vi "INA219 Read Measurements.vi"(8 "error in (no error)":errorcluster, 9 "INA219 Config Options":T1={"I2C"={"Slave Address"=64, "Channel"=0}, "Reset bit"=0, "Bus Voltage Range"=1, "PGA/Shunt Voltage Gain"=3, "Bus Voltage ADC Settings"=8, "Shunt Voltage ADC Settings"=3, "Mode"=7, "Calibration Value"=4096, "Online"=FALSE, "Shunt Resistor"=0.1} {"Shunt Resistor" format="%#_g ohm"; "I2C"."Slave Address" format="%.0x"; "Calibration Value" format="%.0x"; "Mode" items=["Power Down", "Shunt Voltage, Triggered", "Bus Voltage, Triggered", "Shunt & Bus, Triggered", "ADC Off (Disabled)", "Shunt Voltage, Continuous", "Bus Voltage, Continuous", "Shunt & Bus Voltage, Continuous"]; "Shunt Voltage ADC Settings" items=["9-bit, 84us conversion time"=0, "10-bit, 148us conversion time"=1, "11-bit, 276us conversion time"=2, "12-bit, 532us conversion time"=3, "1x12-bit, 532us conversion time"=8, "2x12-bit averaged, 1.06ms conversion time"=9, "4x12-bit averaged, 2.13ms conversion time"=10, "8x12-bit averaged, 4.26ms conversion time"=11, "16x12-bit averaged, 8.51ms conversion time"=12, "32x12-bit averaged, 17.02ms conversion time"=13, "64x12-bit averaged, 34.05ms conversion time"=14, "128x12-bit averaged, 68.10ms conversion time"=15]; "Bus Voltage ADC Settings" items=["9-bit, 84us conversion time"=0, "10-bit, 148us conversion time"=1, "11-bit, 276us conversion time"=2, "12-bit, 532us conversion time"=3, "1x12-bit, 532us conversion time"=8, "2x12-bit averaged, 1.06ms conversion time"=9, "4x12-bit averaged, 2.13ms conversion time"=10, "8x12-bit averaged, 4.26ms conversion time"=11, "16x12-bit averaged, 8.51ms conversion time"=12, "32x12-bit averaged, 17.02ms conversion time"=13, "64x12-bit averaged, 34.05ms conversion time"=14, "128x12-bit averaged, 68.10ms conversion time"=15]; "PGA/Shunt Voltage Gain" items=["Gain 1, +/-40mV", "Gain 2, +/-80mV", "Gain 3, +/-160mV", "Gain 4, +/-320mV"]; "Bus Voltage Range" items=["0-16V Range", "0-32V Range"]; "Reset bit" items=["Do Not Reset", "Reset"]}, 11 "LINX Resource in":T3) -> (0 "error out":errorcluster, 1 "INA219 Config Options":T1={"I2C"={"Slave Address"=64, "Channel"=0}, "Reset bit"=0, "Bus Voltage Range"=1, "PGA/Shunt Voltage Gain"=3, "Bus Voltage ADC Settings"=8, "Shunt Voltage ADC Settings"=3, "Mode"=7, "Calibration Value"=4096, "Online"=FALSE, "Shunt Resistor"=0.1} {"Shunt Resistor" format="%#_g ohm"; "I2C"."Slave Address" format="%.0x"; "Calibration Value" format="%.0x"; "Mode" items=["Power Down", "Shunt Voltage, Triggered", "Bus Voltage, Triggered", "Shunt & Bus, Triggered", "ADC Off (Disabled)", "Shunt Voltage, Continuous", "Bus Voltage, Continuous", "Shunt & Bus Voltage, Continuous"]; "Shunt Voltage ADC Settings" items=["9-bit, 84us conversion time"=0, "10-bit, 148us conversion time"=1, "11-bit, 276us conversion time"=2, "12-bit, 532us conversion time"=3, "1x12-bit, 532us conversion time"=8, "2x12-bit averaged, 1.06ms conversion time"=9, "4x12-bit averaged, 2.13ms conversion time"=10, "8x12-bit averaged, 4.26ms conversion time"=11, "16x12-bit averaged, 8.51ms conversion time"=12, "32x12-bit averaged, 17.02ms conversion time"=13, "64x12-bit averaged, 34.05ms conversion time"=14, "128x12-bit averaged, 68.10ms conversion time"=15]; "Bus Voltage ADC Settings" items=["9-bit, 84us conversion time"=0, "10-bit, 148us conversion time"=1, "11-bit, 276us conversion time"=2, "12-bit, 532us conversion time"=3, "1x12-bit, 532us conversion time"=8, "2x12-bit averaged, 1.06ms conversion time"=9, "4x12-bit averaged, 2.13ms conversion time"=10, "8x12-bit averaged, 4.26ms conversion time"=11, "16x12-bit averaged, 8.51ms conversion time"=12, "32x12-bit averaged, 17.02ms conversion time"=13, "64x12-bit averaged, 34.05ms conversion time"=14, "128x12-bit averaged, 68.10ms conversion time"=15]; "PGA/Shunt Voltage Gain" items=["Gain 1, +/-40mV", "Gain 2, +/-80mV", "Gain 3, +/-160mV", "Gain 4, +/-320mV"]; "Bus Voltage Range" items=["0-16V Range", "0-32V Range"]; "Reset bit" items=["Do Not Reset", "Reset"]}, 2 "Measurements":T2 {"Current" format="%#.3g A"; "Power" format="%#.3g W"; "Shunt Voltage" format=" %#.3g V"; "Bus Voltage" format="%#.3g V"; "Voltage (Total)" format="%#.3g V"}, 3 "LINX Resource":T3)   [LabVIEW 2014]
uses:
  <vilib>/MakerHub/LINX/Private/Type Defs/LINX Ref.ctl
  <vilib>/MakerHub/LINX/Private/Type Defs/Platform.ctl
  <vilib>/MakerHub/LINX/Private/Type Defs/Interface.ctl
  <vilib>/MakerHub/LINX/Private/Device/Type Defs/LINX Device Config.ctl
  <vilib>/MakerHub/LINX/Private/Device/Type Defs/TCP Config.ctl
  <vilib>/MakerHub/LINX/Private/Device/Type Defs/Channels.ctl
  INA219 Measurements.ctl
  INA219 Config Options.ctl
  <vilib>/MakerHub/LINX/LMH-LINX.lvlib
  <vilib>/MakerHub/LINX/Private/Device/Device.lvlib
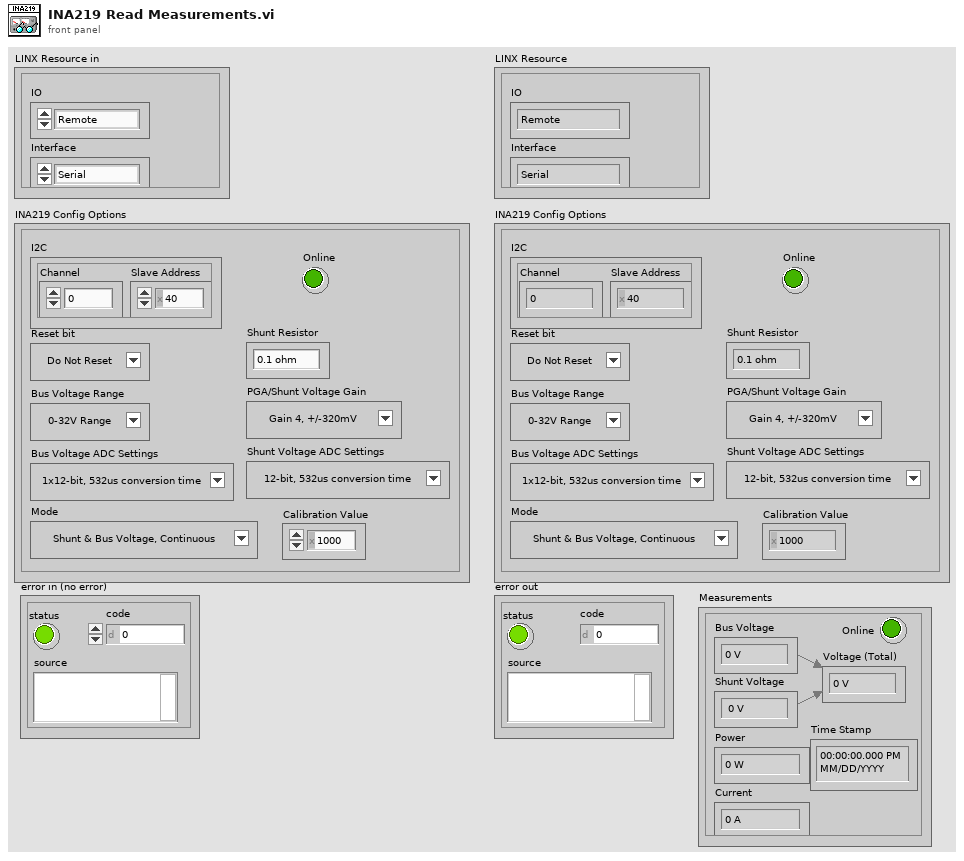
[diagram p1: front panel]
types:
  T1 = typedef "INA219 Config Options.ctl" = cluster{"I2C":cluster{"Slave Address":u8, "Channel":u8}, "Reset bit":u8, "Bus Voltage Range":u8, "PGA/Shunt Voltage Gain":u8, "Bus Voltage ADC Settings":u8, "Shunt Voltage ADC Settings":u8, "Mode":u8, "Calibration Value":u16, "Online":bool, "Shunt Resistor":dbl}
  T2 = typedef "INA219 Measurements.ctl" = cluster{"Voltage (Total)":dbl, "Bus Voltage":dbl, "Shunt Voltage":dbl, "Power":dbl, "Current":dbl, "Online":bool, "Time Stamp":timestamp}
  T3 = typedef "LMH-LINX.lvlib/LINX Ref.ctl" = cluster{"IO":T4, "Interface":T5, "LINX Device Config":T6}
  T4 = typedef "LMH-LINX.lvlib/Platform.ctl" = enum16{"Remote", "Local"}
  T5 = typedef "LMH-LINX.lvlib/Interface.ctl" = enum16{"Serial", "TCP"}
  T6 = typedef "LMH-LINX.lvlib/Device.lvlib/LINX Device Config.ctl" = cluster{"Interface":T5, "COM Port":refnum<visa-resource-name>, "TCP Configuration":T7, "Device Family":u8, "Device ID":u8, "Device Name":string, "TCP Ref":refnum<k5>, "Channels":T8}
  T7 = typedef "LMH-LINX.lvlib/Device.lvlib/TCP Config.ctl" = cluster{"IP Address":string, "Port":u16}
  T8 = typedef "LMH-LINX.lvlib/Channels.ctl" = cluster{"DI":u8[], "DO":u8[], "AI":u8[], "AO":u8[], "PWM":u8[], "QE":u8[], "UART":u8[], "I2C 2":u8[], "SPI":u8[], "CAN":u8[], "Servo":u8[], "AI Ref (V)":dbl, "AI Resolution (Bits)":u8, "AO Ref (V)":dbl, "AO Resolution (Bits)":u8}
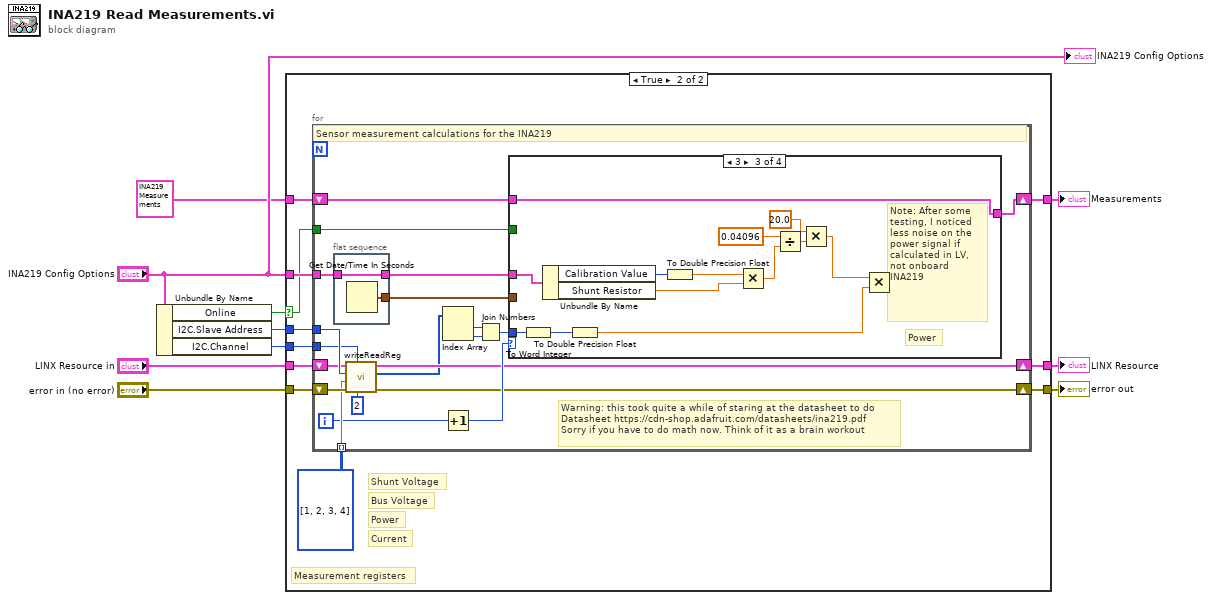
[diagram p0: block diagram]
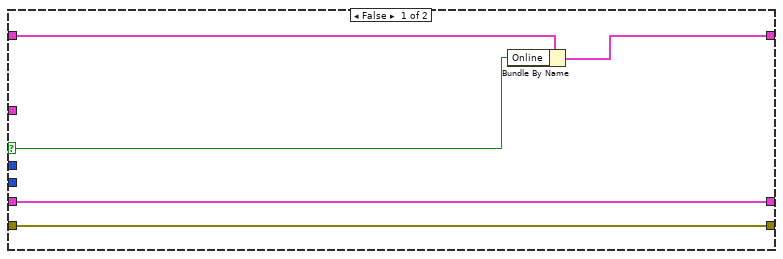
[diagram p2: hidden frame]
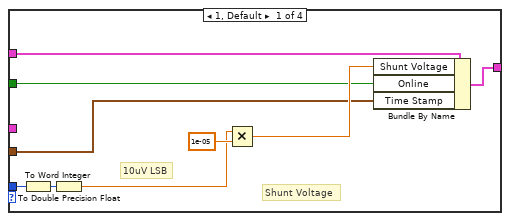
[diagram p3: hidden frame]
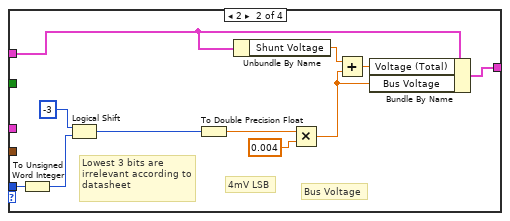
[diagram p4: hidden frame]
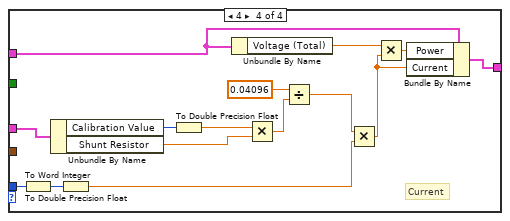
[diagram p5: hidden frame]
diagram:
  n1 = Unbundle By Name("INA219 Config Options") -> ("Online"=w1:bool, "I2C.Slave Address"=w4:u8, "I2C.Channel"=w5:u8)
  n2 = case shown="True" w1 {
    selector: w1 -> [w11 w16]
    tunnel: "error in (no error)" -> [w14 w26]
    tunnel: "LINX Resource in" -> [w15 w25]
    tunnel: [w14 w24] -> w8
    tunnel: [w15 w23] -> w7
    tunnel: [w12 w21] -> w6
    tunnel: w5 -> [_ w20]
    tunnel: w4 -> [_ w19]
    tunnel: "INA219 Config Options" -> [_ w18]
    tunnel: T2 {"Voltage (Total)"=0.0, "Bus Voltage"=0.0, "Shunt Voltage"=0.0, "Power"=0.0, "Current"=0.0, "Online"=FALSE, "Time Stamp"=timestamp(0 s since 1904-01-01)} ("Measurements") -> [w13 w17]
    frame False {
      n3 = Bundle By Name(cluster=w13, "Online"=w11) -> (w12:T2)
    }
    frame True {
      # "Measurement registers"
      # "Current"
      # "Power"
      # "Bus Voltage"
      # "Shunt Voltage"
      n4 = for {
        tunnel: w19 -> [w46]
        tunnel: w20 -> [w45]
        shift-right: [w32] -> w24
        shift-left: w26 -> [w44]
        shift-right: [w33] -> w23
        shift-left: w25 -> [w43]
        tunnel: u8[][] [[1], [2], [3], [4]] ("Data") -> [w42] mode=indexing
        tunnel: w18 -> [w29]
        shift-right: [w35] -> w21
        shift-left: w17 -> [w36]
        tunnel: w16 -> [w30]
        i -> [w39]
        # "Warning: this took quite a while of staring at the datasheet to do\nDatasheet https://cdn-shop.adafruit.com/datasheets/ina219.pdf\nSorry if you have to do math now. Think of it as a brain workout"
        # "Sensor measurement calculations for the INA219"
        n5 = flat-sequence {
          tunnel: w29 -> [w48]
          tunnel: [w48] -> w28
          tunnel: [w47] -> w27
          frame #0 {
            n6 = Get Date/Time In Seconds() -> (seconds since 1Jan1904=w47:timestamp)
          }
        }
        n7 = call "writeReadReg.vi"("Bytes To Read"=u8 2, "I2C Channel"=w45, "error in"=w44, "Data"=w42, "I2C Slave Address"=w46, "LINX Resource in"=w43) -> ("error out"=w32:errorcluster, "Bytes Read"=w31:u8[], "LINX Resource out"=w33:T3)  [unwired: 3 in]
        n8 = Index Array(array=w31) -> (element #1=w40:u8, element #2=w41:u8)  [unwired: 2 in]
        n9 = Increment(x=w39) -> (x+1=w38:i32)
        n10 = Join Numbers(hi=w40, lo=w41) -> ((hi.lo)=w37:u16)
        n11 = case shown="3" w38 {
          tunnel: w37 -> [w56 w62 w80 w95]
          tunnel: w28 -> [_ _ w81 w96]
          tunnel: w36 -> [w57 w67 w70 w86]
          tunnel: [w53 w68 w70 w93] -> w35
          tunnel: w30 -> [w50 _ _ _]
          tunnel: w27 -> [w49 _ _ _]
          frame 1, Default {
            # "10uV LSB"
            # "Shunt Voltage"
            n12 = To Word Integer(number=w56) -> (16bit integer=w54:i16)
            n13 = To Double Precision Float(number=w54) -> (double precision float=w51:dbl)
            n14 = Multiply(x=w51, y=1e-05) -> (x*y=w55:dbl)
            n15 = Bundle By Name(cluster=w57, "Shunt Voltage"=w55, "Online"=w50, "Time Stamp"=w49) -> (w53:T2)
          }
          frame 2 {
            # "Lowest 3 bits are irrelevant according to datasheet"
            # "4mV LSB"
            # "Bus Voltage"
            n16 = To Unsigned Word Integer(number=w62) -> (unsigned 16bit integer=w61:u16)
            n17 = Logical Shift(y=i16 -3, x=w61) -> (x << y=w59:u16)
            n18 = To Double Precision Float(number=w59) -> (double precision float=w63:dbl)
            n19 = Unbundle By Name(w67) -> ("Shunt Voltage"=w65:dbl)
            n20 = Multiply(x=w63, y=0.004) -> (x*y=w66:dbl)
            n21 = Add(x=w65, y=w66) -> (x+y=w58:dbl)
            n22 = Bundle By Name(cluster=w67, "Voltage (Total)"=w58, "Bus Voltage"=w66) -> (w68:T2)
          }
          frame 3 {
            # "Note: After some testing, I noticed less noise on the power signal if calculated in LV, not onboard INA219"
            # "Power"
            n23 = To Word Integer(number=w80) -> (16bit integer=w75:i16)
            n24 = Unbundle By Name(w81) -> ("Calibration Value"=w76:u16, "Shunt Resistor"=w69:dbl)
            n25 = To Double Precision Float(number=w75) -> (double precision float=w74:dbl)
            n26 = To Double Precision Float(number=w76) -> (double precision float=w77:dbl)
            n27 = Multiply(x=w77, y=w69) -> (x*y=w79:dbl)
            n28 = Divide(x=0.04096, y=w79) -> (x/y=w72:dbl)
            n29 = Multiply(x=20.0, y=w72) -> (x*y=w73:dbl)
            n30 = Multiply(x=w73, y=w74) -> ()  [unwired: 1 out]
          }
          frame 4 {
            # "Current"
            n31 = To Word Integer(number=w95) -> (16bit integer=w94:i16)
            n32 = Unbundle By Name(w96) -> ("Calibration Value"=w90:u16, "Shunt Resistor"=w82:dbl)
            n33 = To Double Precision Float(number=w94) -> (double precision float=w88:dbl)
            n34 = To Double Precision Float(number=w90) -> (double precision float=w89:dbl)
            n35 = Unbundle By Name(w86) -> ("Voltage (Total)"=w84:dbl)
            n36 = Multiply(x=w89, y=w82) -> (x*y=w92:dbl)
            n37 = Divide(x=0.04096, y=w92) -> (x/y=w87:dbl)
            n38 = Multiply(x=w87, y=w88) -> (x*y=w85:dbl)
            n39 = Multiply(x=w84, y=w85) -> (x*y=w83:dbl)
            n40 = Bundle By Name(cluster=w86, "Power"=w83, "Current"=w85) -> (w93:T2)
          }
        }
      }
    }
  }
  "error out" <- w8
  "LINX Resource" <- w7
  "Measurements" <- w6
  "INA219 Config Options" <- "INA219 Config Options"
